vi "Send Test Number.vi"() -> (0 "error out":errorcluster)   [LabVIEW 2020]
uses:
  <vilib>/IlluminatedG/lv-stream/stream/Stream.lvclass/Stream.ctl
  <vilib>/IlluminatedG/lv-stream/stream/Dispatch Sniffer Data.vi
  <vilib>/IlluminatedG/lv-stream/stream/Prepared.vi
  <vilib>/IlluminatedG/lv-stream/Endpoint/Cast Sniffer Callback.vi
  Stream-Websocket/WebsocketStream/WebsocketStream.lvclass
  C:/Program Files (x86)/National Instruments/LabVIEW 2020/vi.lib/IlluminatedG/lv-stream/stream/Stream.lvclass
  <vilib>/Utility/error.llb/Error Cluster From Error Code.vi
  <vilib>/IlluminatedG/lv-stream/stream/Stream.lvclass
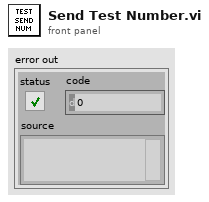
[diagram p1: front panel]
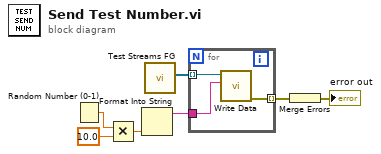
[diagram p0: block diagram]
diagram:
  n1 = Random Number (0-1)() -> (number: 0 to 1=w6:dbl)
  n2 = Multiply(x=w6, y=10.0) -> (x*y=w4:dbl)
  n3 = Format Into String(w4) -> (resulting string=w3:string)  [unwired: 3 in, 1 out]
  n4 = call "Test Streams FG.vi"() -> ("Streams"=w7:refnum<class "WebsocketStream.lvclass">[])  [unwired: 11 in]
  n5 = for {
    tunnel: w7 -> [w10] mode=indexing
    tunnel: w3 -> [w9]
    tunnel: [w8] -> w2 mode=indexing
    n6 = call <vilib>:"Write Data.vi"("Data"=w9, "Stream in"=w10) -> ("error out"=w8:errorcluster)  [unwired: 8 in, 1 out]
  }
  n7 = Merge Errors(w2) -> (→"error out":errorcluster)
